vi "ABB Calc NL loss.vi"(1 "SR95":dbl, 2 "No load test results 2":dbl[][](array[numeric])) -> (0 "No load test results":dbl[][](array[numeric]))   [LabVIEW 2017]
uses:
  <vilib>/Analysis/NI_AALPro.lvlib
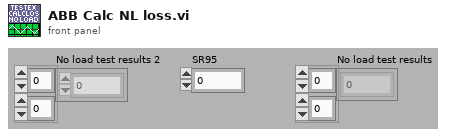
[diagram p1: front panel]
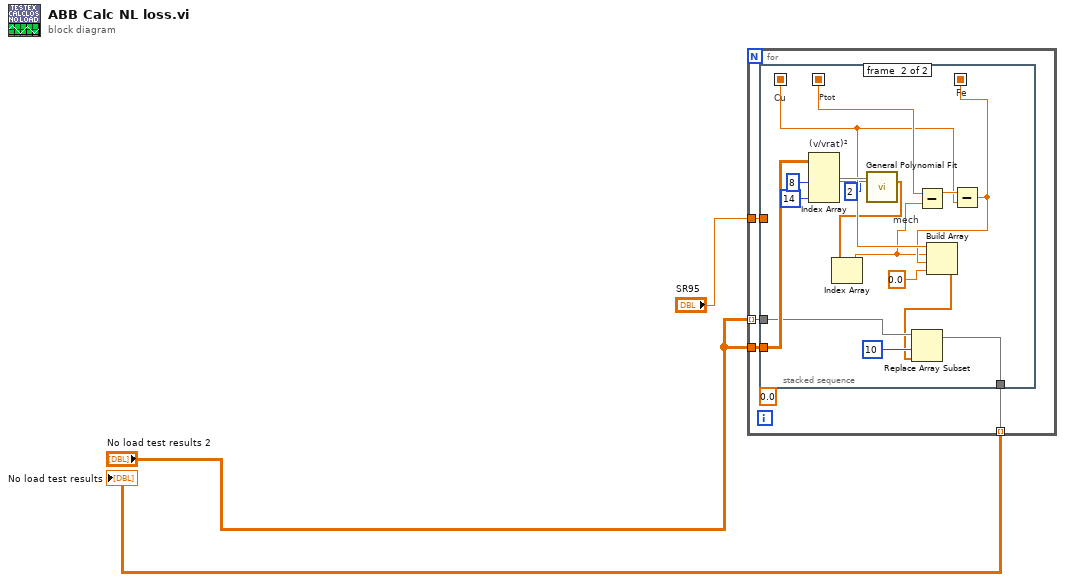
[diagram p0: block diagram]
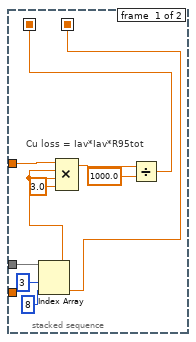
[diagram p2: hidden frame]
diagram:
  n1 = for {
    tunnel: "No load test results 2" -> [w6] mode=indexing
    tunnel: "SR95" -> [w7]
    tunnel: "No load test results 2" -> [w5]
    tunnel: [w4] -> w3 mode=indexing
    (unwired) 0.0 ("Numeric")
    n2 = stacked-sequence {
      seq-local: [w10 _] -> [_ w27]
      seq-local: [w11 _] -> [_ w34]
      seq-local: [_ w26] -> [_ _]
      tunnel: w7 -> [w17 _]
      tunnel: w6 -> [w14 w28]
      tunnel: w5 -> [_ w32]
      tunnel: [_ w23] -> w4
      frame #0 {
        # "Cu loss = Iav*Iav*R95tot"
        n3 = Index Array(array=w14, index #1=3 ("index"), index #2=8 ("index")) -> (element #1=w9:dbl, element #2=w11:dbl)
        n4 = Compound Arithmetic op=MULTIPLY(w17, w9, w9, 3.0 ("value")) -> (w16:dbl)
        n5 = Divide(x=w16, y=1000.0) -> (x/y=w10:dbl)
      }
      frame #1 {
        # "mech"
        # "Fe"
        # "Ptot"
        # "Cu"
        n6 = Index Array "(v/vrat)²"(array=w32, index (col) #1=8 ("disabled index (col)"), index (col) #2=14 ("index (col)")) -> (element #1=w31:dbl[], element #2=w22:dbl[])  [unwired: 2 in]
        n7 = call <vilib>:"General Polynomial Fit.vi"("Y"=w31, "polynomial order"=2, "X"=w22) -> ("Polynomial Coefficients"=w19:dbl[])  [unwired: 9 in, 3 out]
        n8 = Index Array(array=w19) -> (element=w18:dbl)  [unwired: 1 in]
        n9 = Subtract(x=w34, y=w18) -> (x-y=w33:dbl)
        n10 = Subtract(x=w33, y=w27) -> (x-y=w26:dbl)
        n11 = Build Array(w27, w18, w26, 0.0 ("element")) -> (w24:dbl[])
        n12 = Replace Array Subset(array=w28, new element=w24, index=10) -> (w23:dbl[])
      }
    }
  }
  "No load test results" <- w3
